vi "autoinfo.vi"() -> ()   [LabVIEW 2019]
panel:
  out "Auto_Test_Heading (deg)":dbl format="%#_13g"
  out "Auto_Error":errorcluster
  out "Distance_From_Start (in)":dbl
  out "Distance_From_End (in)":dbl
  out "Auto_Subsystem_Step":i32
  out "Auto_Drive_Step":i32
  out "Auto_Subsystem_Action":string
  out "Auto_Drive_Action":string
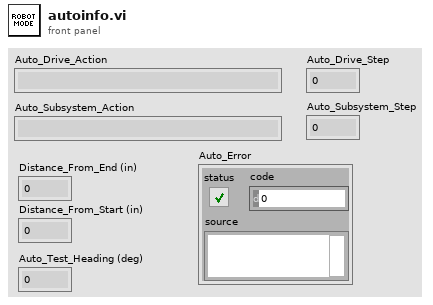
[diagram p1: front panel]
diagram:
